vi "String to Double.vi"(7 "use system decimal point (T)":bool, 11 "fractionalString":string) -> (3 "value":dbl)   [LabVIEW 2018]
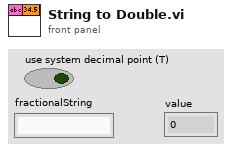
[diagram p1: front panel]
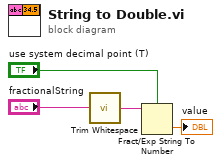
[diagram p0: block diagram]
diagram:
  n1 = call <vilib>:"Trim Whitespace.vi"("string"="fractionalString") -> ("trimmed string"=w3:string)  [unwired: 1 in]
  n2 = Fract/Exp String To Number(use system decimal point (T)="use system decimal point (T)", string=w3) -> (number=→"value":dbl)  [unwired: 2 in, 1 out]
